vi "Close.vi"(8 "error in (no error)":errorcluster, 11 "C4209 PNA":refnum<class "C4209 PNA.lvclass">) -> (0 "error out":errorcluster, 3 "C4209 PNA out":refnum<class "C4209 PNA.lvclass">)   [LabVIEW 2017, in "C4209 PNA.lvclass"]
uses:
  C4209 PNA.lvclass
  C4209 PNA.lvclass/C4209 PNA.ctl
  <instrlib>/CMT S2 Series VNA/CMT S2 Series VNA.lvlib
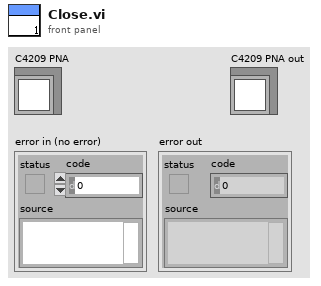
[diagram p1: front panel]
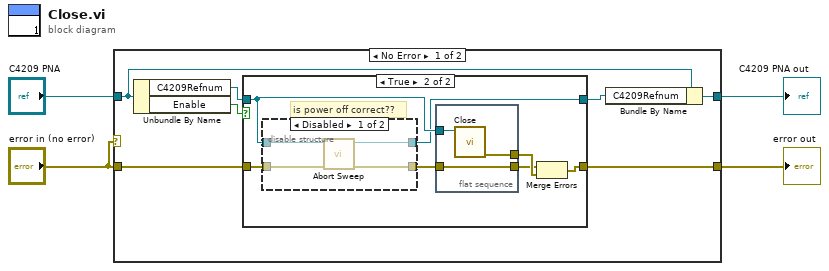
[diagram p0: block diagram]
diagram:
  n1 = case shown="No Error" "error in (no error)" {
    tunnel: "C4209 PNA" -> [w6 w30]
    tunnel: [w10 w31] -> w3
    tunnel: "error in (no error)" -> [w9 w31]
    tunnel: [w8 w30] -> w2
    frame No Error {
      n2 = Unbundle By Name(w6) -> ("C4209Refnum"=w11:refnum<k7>, "Enable"=w7:bool)
      n3 = case shown="True" w7 {
        tunnel: w11 -> [w12 w15]
        tunnel: w9 -> [w13 w20]
        tunnel: [w13 w18] -> w10
        tunnel: [w12 w14] -> w5
        frame False {
        }
        frame True {
          # "is power off correct??"
          n4 = disable-structure shown="Disabled" {
            disable-tunnel: w20 -> [w22 w26]
            disable-tunnel: [w21 w26] -> w17
            disable-tunnel: w15 -> [w24 w25]
            disable-tunnel: [w23 w25] -> w14
            frame Disabled {
              n5 = call <instrlib>:"Abort Sweep.vi"("error in (no error)"=w22, "Reference in"=w24) -> ("error out"=w21:errorcluster, "Reference out"=w23:refnum<k7>)  [unwired: 8 in]
            }
            frame Enabled {
            }
          }
          n6 = flat-sequence {
            tunnel: w15 -> [w27]
            tunnel: [w28] -> w19
            tunnel: [w29] -> w16
            tunnel: w17 -> [w29]
            frame #0 {
              n7 = call <instrlib>:"Close.vi"("Reference in"=w27) -> ("error out"=w28:errorcluster)  [unwired: 10 in]
            }
          }
          n8 = Merge Errors(w16, w19) -> (w18:errorcluster)
        }
      }
      n9 = Bundle By Name(cluster=w6, "C4209Refnum"=w5) -> (w8:refnum<class "C4209 PNA.lvclass">)
    }
    frame Error {
    }
  }
  "error out" <- w3
  "C4209 PNA out" <- w2
